vi "ProScan 3 Check Range.vi"(0 "Setpoint":dbl[](array[numeric]), 2 "Range Limit":dbl=0.02, 11 "Position":dbl[](array[numeric])) -> (8 "In Range?":bool)   [LabVIEW 2016]
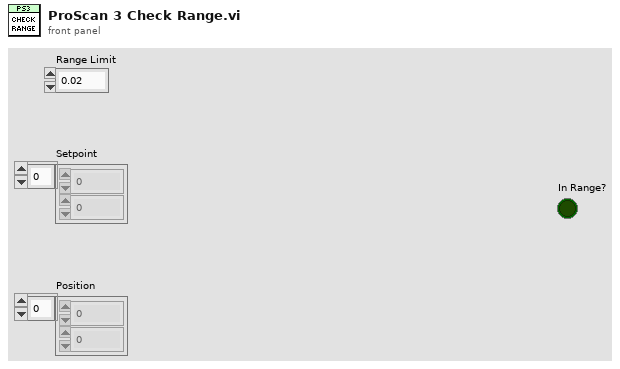
[diagram p1: front panel]
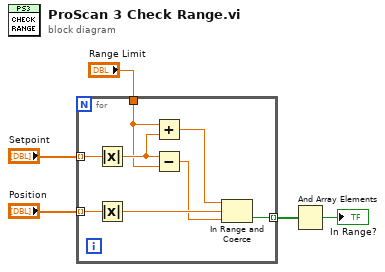
[diagram p0: block diagram]
diagram:
  n1 = for {
    tunnel: "Setpoint" -> [w12] mode=indexing
    tunnel: "Position" -> [w11] mode=indexing
    tunnel: [w10] -> w3 mode=indexing
    tunnel: "Range Limit" -> [w8]
    n2 = Absolute Value(x=w12) -> (abs(x)=w9:dbl)
    n3 = Absolute Value(x=w11) -> (abs(x)=w13:dbl)
    n4 = Add(x=w8, y=w9) -> (x+y=w6:dbl)
    n5 = Subtract(x=w9, y=w8) -> (x-y=w7:dbl)
    n6 = In Range and Coerce(upper limit=w6, x=w13, lower limit=w7) -> (In Range?=w10:bool)  [unwired: 1 out]
  }
  n7 = And Array Elements(Boolean array=w3) -> (logical AND=→"In Range?":bool)
